vi "PH_GUI.set U16 GUI object.vi"(2 "U16 Ref":refnum<vi>, 3 "Value":u16, 4 "Blinking (false)":bool, 5 "error in (no error)":errorcluster) -> (19 "error out":errorcluster)   [LabVIEW 2014, in "PH_Common.lvlib"]
doc: "Sets value and more for the referenced GUI object."
uses:
  PH_Common.lvlib
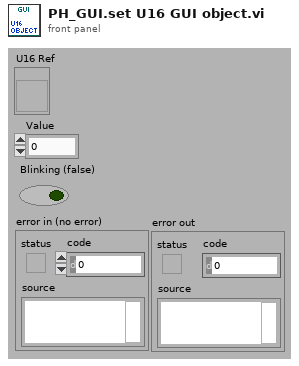
[diagram p1: front panel]
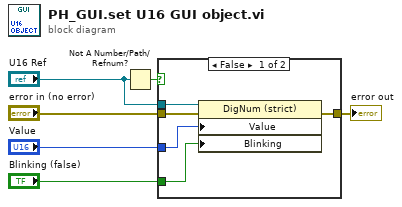
[diagram p0: block diagram]
diagram:
  n1 = Not A Number/Path/Refnum?(number/path/refnum="U16 Ref") -> (NaN/Path/Refnum?=w5:bool)
  n2 = case shown="False" w5 {
    tunnel: "error in (no error)" -> [w7 w12]
    tunnel: "U16 Ref" -> [w8 _]
    tunnel: "Value" -> [w9 _]
    tunnel: "Blinking (false)" -> [w10 _]
    tunnel: [w11 w12] -> w2
    frame False {
      n3 = property class="DigNum (strict)"(reference=w8, error in=w7, "Value"=w9, "Blinking"=w10) -> (error out=w11:errorcluster)  [unwired: 1 out]
    }
    frame True {
    }
  }
  "error out" <- w2
